vi "Compare String by Regular Expression.vi"(8 "error in":errorcluster, 10 "regular expression":string, 11 "String":string) -> (0 "error out":errorcluster, 3 "x = y?":bool)   [LabVIEW 2021, in "CANOpen Addon System Explorer.lvlib"]
uses:
  CANOpen Addon System Explorer.lvlib
  <vilib>/regexp/Match Regular Expression.xnode
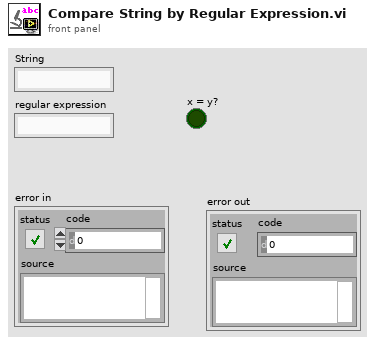
[diagram p1: front panel]
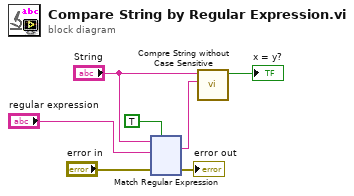
[diagram p0: block diagram]
diagram:
  n1 = xnode "Match Regular Expression"("input string"="String", "regular expression"="regular expression", "error in"="error in", "ignore case? (F)"=TRUE) -> ("whole match"=w2:string, "error out"=→"error out":errorcluster)  [unwired: 2 in, 3 out]
  n2 = call "Compre String without Case Sensitive .vi"("String B"=w2, "String A"="String") -> ("A=B?"=→"x = y?":bool)  [unwired: 9 in]
